vi "VRM_query.vi"() -> ()   [LabVIEW 2019]
uses:
  <instrlib>/Mercury iXX/Public/Libraries/Magnet/Controls/Identifier.ctl
  <instrlib>/Mercury iXX/Public/Controls/Response String.ctl
  <instrlib>/Mercury iXX/Public/Libraries/Magnet/Controls/PSU Actions.ctl
  <instrlib>/Mercury iXX/Public/Controls/Comms Transport Layer.ctl
  <instrlib>/Mercury iXX/Public/Libraries/System/Open/Open System.vi
  <instrlib>/Mercury iXX/Public/Libraries/System/Read/Catalogue (Read).vi
  <instrlib>/Mercury iXX/Mercury iXX.lvlib
  <instrlib>/Mercury iXX/Public/Libraries/Magnet/Open/Open Magnet Device.vi
  <instrlib>/Mercury iXX/Public/Libraries/Magnet.lvlib
  <instrlib>/Mercury iXX/Public/Libraries/Magnet/Signals/Read/Current (Read).vi
  <instrlib>/Mercury iXX/Public/Libraries/System.lvlib
  <instrlib>/Mercury iXX/Public/Libraries/Magnet/Configuration/Set/PSU Action Status (Set).vi
  <instrlib>/Mercury iXX/Public/Libraries/Magnet/Signals/Set/Target Field Rate (Set).vi
  <instrlib>/Mercury iXX/Public/Libraries/Magnet/Signals/Set/Target Field (Set).vi
  <instrlib>/Mercury iXX/Public/Libraries/Magnet/Configuration/Read/PSU Action Status (Read).vi
  <instrlib>/Mercury iXX/Public/Libraries/Magnet/Signals/Read/Field (Read).vi
panel:
  out "PSU Act Stat":T1 caption="PSU Action Status"
  in  "stop":bool
  out "error out":errorcluster
  out "Response 2":T2
  out "Response":T2
  in  "Target Field":dbl format="%#.2f"
  out "Read 1":dbl
  in  "Device ID 3":string(combo)="PSU.M1"
  in  "Device ID 2":string(combo)="GRPY"
  in  "Device ID 1":T3="GRPZ"
  out "Read 2":dbl format="%_15p"
  out "Read 3":dbl format="%_10p"
  out "Devices":string[](array[string])
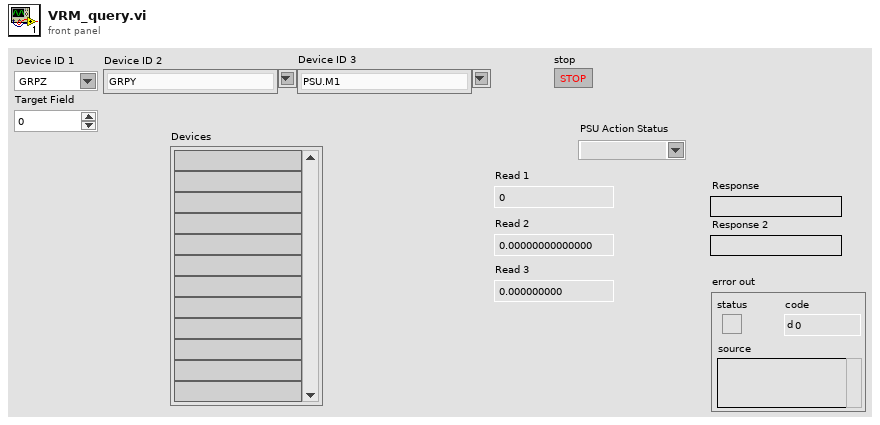
[diagram p1: front panel]
types:
  T1 = typedef "Mercury iXX.lvlib/Magnet.lvlib/PSU Actions.ctl" = string
  T2 = typedef "Mercury iXX.lvlib/Response String.ctl" = string
  T3 = typedef "Mercury iXX.lvlib/Magnet.lvlib/Identifier.ctl" = string
  T4 = typedef "Mercury iXX.lvlib/Comms Transport Layer.ctl" = enum16{"Ethernet TCP/IP", "USB", "ISOBus - RS-232", "GPIB"}
  T5 = typedef "Mercury iXX.lvlib/Mercury Reference.ctl" = cluster{"Comms":refnum<visa-resource-name>, "Device ID":string[], "Comms Layer":T4, "Command":string, "Query reference":T6}
  T6 = typedef "Mercury iXX.lvlib/Query Dynamic Reference.ctl" = refnum<vi>
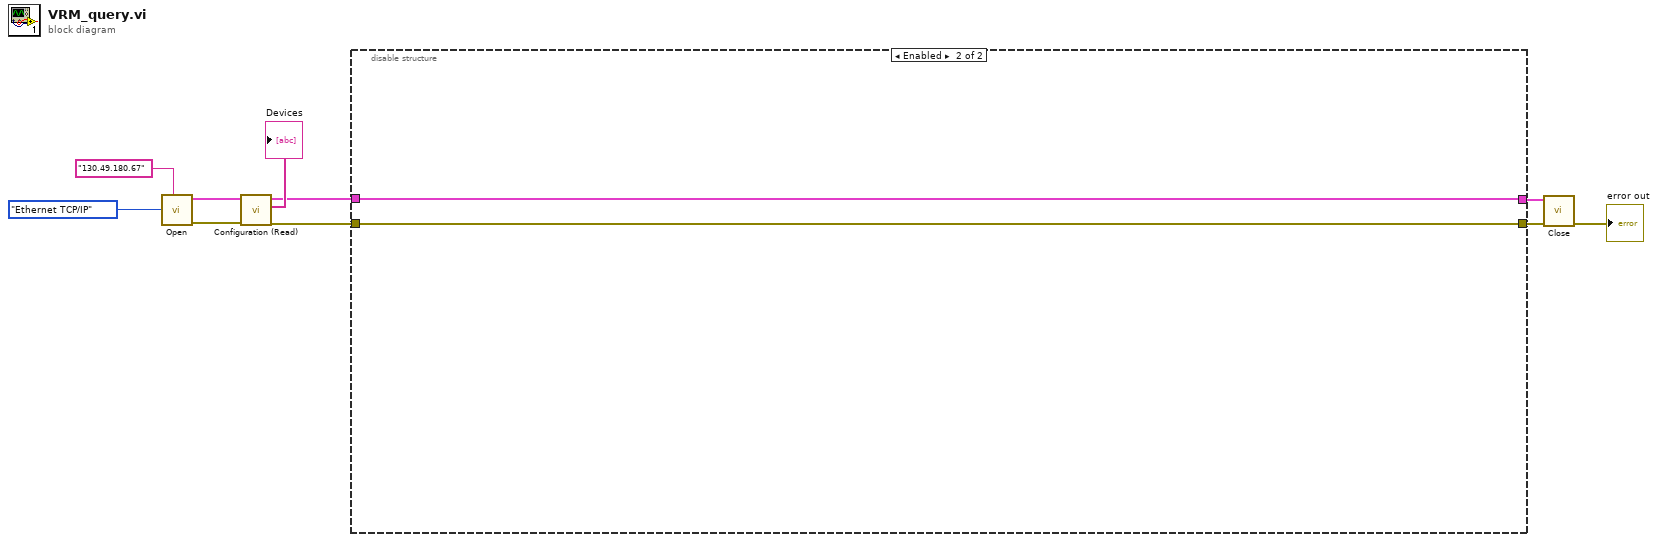
[diagram p0: block diagram]
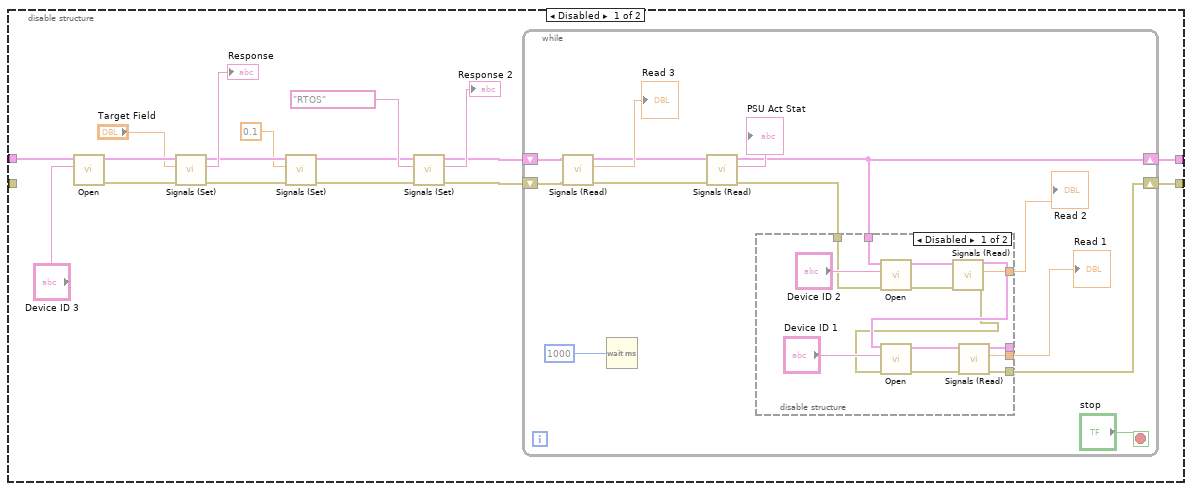
[diagram p2: hidden frame]
diagram:
  n1 = call-poly <instrlib>:"Open.vi"("IP Address"="130.49.180.67", "Comms Layer"=Comms_Transport_Layer."Ethernet TCP/IP") -> ("error out"=w7:errorcluster, "Mercury Reference Out"=w8:T5)  [unwired: 5 in, 3 out]
  n2 = call-poly <instrlib>:"Configuration (Read).vi"("error in"=w7, "Mercury Reference In"=w8) -> ("error out"=w1:errorcluster, "Devices"=→"Devices":string[], "Mercury Reference Out"=w5:T5)  [unwired: 6 in, 1 out]
  n3 = disable-structure shown="Enabled" {
    disable-tunnel: w5 -> [w26 w56]
    disable-tunnel: [w12 w56] -> w3
    disable-tunnel: [w11 w55] -> w2
    disable-tunnel: w1 -> [_ w55]
    frame Disabled {
      n4 = call-poly <instrlib>:"Open.vi"("Device Identifier"="Device ID 3", "Mercury Reference In"=w26) -> ("error out"=w23:errorcluster, "Mercury Reference Out"=w25:T5)  [unwired: 8 in]
      n5 = call-poly <instrlib>:"Signals (Set).vi"("error in"=w23, "Target Field"="Target Field", "Mercury Reference In"=w25) -> ("error out"=w13:errorcluster, "Response"=→"Response":T2, "Mercury Reference Out"=w17:T5)  [unwired: 5 in, 1 out]
      n6 = call-poly <instrlib>:"Signals (Set).vi"("error in"=w13, "Target Field Rate"=0.1 ("Target Field"), "Mercury Reference In"=w17) -> ("error out"=w14:errorcluster, "Mercury Reference Out"=w15:T5)  [unwired: 5 in, 2 out]
      n7 = call-poly <instrlib>:"Signals (Set).vi"("error in"=w14, "PSU Act Stat"=T1 "RTOS", "Mercury Reference In"=w15) -> ("error out"=w18:errorcluster, "Response"=→"Response 2":T2, "Mercury Reference Out"=w20:T5)  [unwired: 5 in, 1 out]
      n8 = while {
        shift-right: [w28] -> w12
        shift-left: w20 -> [w37]
        shift-right: [w32] -> w11
        shift-left: w18 -> [w36]
        stop <- "stop" stop-if-true
        n9 = call-poly <instrlib>:"Signals (Read).vi"("error in"=w36, "Mercury Reference In"=w37) -> ("error out"=w34:errorcluster, "Field"=→"Read 3":dbl, "Mercury Reference Out"=w33:T5)  [unwired: 5 in, 2 out]
        n10 = Wait (ms)(milliseconds to wait=u32 1000) -> ()  [unwired: 1 out]
        n11 = call-poly <instrlib>:"Signals (Read).vi"("error in"=w34, "Mercury Reference In"=w33) -> ("error out"=w31:errorcluster, "PSU Act Stat"=→"PSU Act Stat":T1, "Mercury Reference Out"=w28:T5)  [unwired: 6 in, 1 out]
        n12 = disable-structure shown="Disabled" {
          disable-tunnel: [w52 _] -> w40
          disable-tunnel: [w48 _] -> w38
          disable-tunnel: w28 -> [w46 _]
          disable-tunnel: [w44 _] -> _
          disable-tunnel: [w43 _] -> w32
          disable-tunnel: w31 -> [w41 _]
          frame Disabled {
            n13 = call-poly <instrlib>:"Open.vi"("error in (no error)"=w41, "Device Identifier"="Device ID 2", "Mercury Reference In"=w46) -> ("error out"=w53:errorcluster, "Mercury Reference Out"=w54:T5)  [unwired: 7 in]
            n14 = call-poly <instrlib>:"Signals (Read).vi"("error in"=w53, "Mercury Reference In"=w54) -> ("error out"=w42:errorcluster, "Current"=w52:dbl, "Mercury Reference Out"=w45:T5)  [unwired: 5 in, 2 out]
            n15 = call-poly <instrlib>:"Open.vi"("error in (no error)"=w42, "Device Identifier"="Device ID 1", "Mercury Reference In"=w45) -> ("error out"=w47:errorcluster, "Mercury Reference Out"=w49:T5)  [unwired: 7 in]
            n16 = call-poly <instrlib>:"Signals (Read).vi"("error in"=w47, "Mercury Reference In"=w49) -> ("error out"=w43:errorcluster, "Current"=w48:dbl, "Mercury Reference Out"=w44:T5)  [unwired: 5 in, 2 out]
          }
          frame Enabled {
          }
        }
        "Read 2" <- w40
        "Read 1" <- w38
      }
    }
    frame Enabled {
    }
  }
  n17 = call <instrlib>:"Close.vi"("error in (no error)"=w2, "Mercury Reference"=w3) -> ("error out"=→"error out":errorcluster)  [unwired: 9 in]
